vi "macro_CallbackHelp_MatrixPlus.vi"   [LabVIEW 2019, in "Trajectory_Library.lvlib"]
uses:
  Trajectory_Library.lvlib
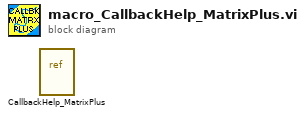
[diagram p0: block diagram]
diagram:
  n1 = vi-ref "CallbackHelp_MatrixPlus.vi"() -> ()  [unwired: 1 out]
